vi "test_SessionsUnregistered_ReserveSessions_IndicatesSessionsDoNotExist.vi"(8 "error in":errorcluster) -> (0 "error out":errorcluster, 2 "result":string, 3 "pass":bool)   [LabVIEW 2020, in "MeasurementServerTests.lvlib" / "Session Reservation Tests.lvlib"]
uses:
  Session Reservation Tests.lvlib
  MeasurementServerTests.lvlib
  Runtime/Measurement Plugin Session Management V1/Session Reservation/Session Reservation.lvclass
  Runtime/Measurement Plugin Session Management Client/RPC Messages/ni_measurementlink_PinMapContext.ctl
  Runtime/Measurement Plugin Session Management Client/Measurement Plugin Session Management Client.lvlib
  Helpers/Pin Map XML Strings Global.vi
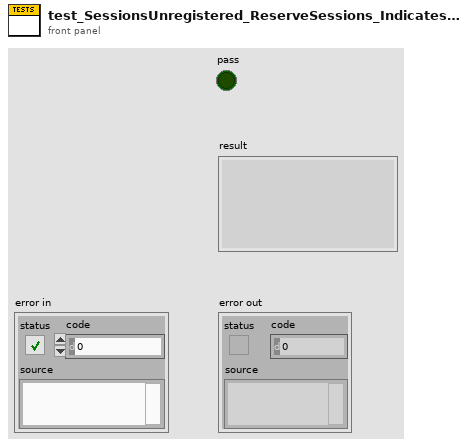
[diagram p1: front panel]
types:
  T1 = typedef "Measurement Plugin Session Management Client.lvlib/ni_measurementlink_PinMapContext.ctl" = cluster{"pin_map_id":string, "sites":i32[]}
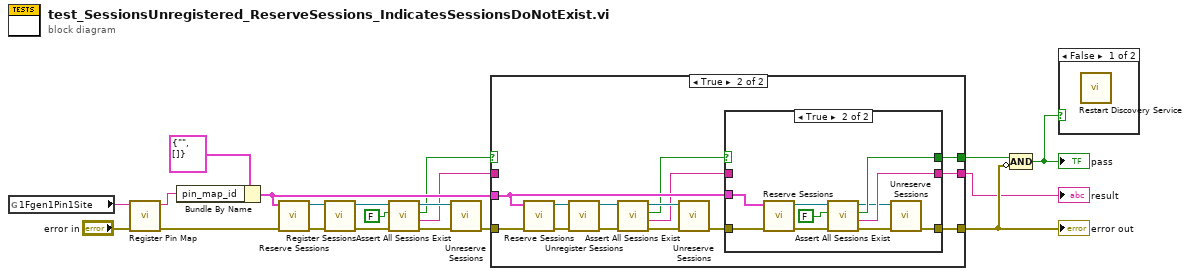
[diagram p0: block diagram]
diagram:
  n1 = global read "Pin Map XML Strings Global.vi" "1Fgen1Pin1Site"() -> (w17:string)
  n2 = call "Register Pin Map.vi"("error in"="error in", "pin map xml"=w17) -> ("error out"=w20:errorcluster, "pin map id"=w18:string)  [unwired: 8 in]
  n3 = Bundle By Name(cluster=T1 {"pin_map_id"="", "sites"=[]} ("pin map context"), "pin_map_id"=w18) -> (w10:T1)
  n4 = call "Reserve Sessions.vi"("error in"=w20, "pin map context"=w10) -> ("error out"=w15:errorcluster, "session reservation out"=w14:refnum<class "Session Reservation.lvclass">)  [unwired: 8 in]
  n5 = call "Register Sessions.vi"("error in"=w15, "session reservation in"=w14) -> ("error out"=w9:errorcluster, "session reservation out"=w7:refnum<class "Session Reservation.lvclass">)  [unwired: 8 in]
  n6 = call "Assert All Sessions Exist.vi"("error in"=w9, "expected value"=FALSE, "session reservation in"=w7) -> ("error out"=w8:errorcluster, "result"=w3:string, "pass"=w4:bool, "session reservation out"=w6:refnum<class "Session Reservation.lvclass">)  [unwired: 5 in]
  n7 = call "Unreserve Sessions.vi"("error in"=w8, "session reservation in"=w6) -> ("error out"=w11:errorcluster)  [unwired: 9 in]
  n8 = case shown="True" w4 {
    selector: w4 -> [w22 _]
    tunnel: [w23 w37] -> w13
    tunnel: w11 -> [w23 w36]
    tunnel: w10 -> [_ w35]
    tunnel: [w22 w25] -> w2
    tunnel: [w21 w24] -> w1
    tunnel: w3 -> [w21 _]
    frame False {
    }
    frame True {
      n9 = call "Reserve Sessions.vi"("error in"=w36, "pin map context"=w35) -> ("error out"=w34:errorcluster, "session reservation out"=w33:refnum<class "Session Reservation.lvclass">)  [unwired: 8 in]
      n10 = call "Unregister Sessions.vi"("error in"=w34, "session reservation in"=w33) -> ("error out"=w31:errorcluster, "session reservation out"=w29:refnum<class "Session Reservation.lvclass">)  [unwired: 8 in]
      n11 = call "Assert All Sessions Exist.vi"("error in"=w31, "session reservation in"=w29) -> ("error out"=w30:errorcluster, "result"=w26:string, "pass"=w27:bool, "session reservation out"=w28:refnum<class "Session Reservation.lvclass">)  [unwired: 6 in]
      n12 = call "Unreserve Sessions.vi"("error in"=w30, "session reservation in"=w28) -> ("error out"=w32:errorcluster)  [unwired: 9 in]
      n13 = case shown="True" w27 {
        selector: w27 -> [w40 _]
        tunnel: [w38 w50] -> w37
        tunnel: w35 -> [_ w49]
        tunnel: w32 -> [w38 w48]
        tunnel: w26 -> [w39 _]
        tunnel: [w40 w44] -> w25
        tunnel: [w39 w43] -> w24
        frame False {
        }
        frame True {
          n14 = call "Reserve Sessions.vi"("error in"=w48, "pin map context"=w49) -> ("error out"=w47:errorcluster, "session reservation out"=w46:refnum<class "Session Reservation.lvclass">)  [unwired: 8 in]
          n15 = call "Assert All Sessions Exist.vi"("error in"=w47, "expected value"=FALSE, "session reservation in"=w46) -> ("error out"=w41:errorcluster, "result"=w43:string, "pass"=w44:bool, "session reservation out"=w42:refnum<class "Session Reservation.lvclass">)  [unwired: 5 in]
          n16 = call "Unreserve Sessions.vi"("error in"=w41, "session reservation in"=w42) -> ("error out"=w50:errorcluster)  [unwired: 9 in]
        }
      }
    }
  }
  "error out" <- w13
  "result" <- w1
  n17 = Compound Arithmetic op=AND(w2, invert w13) -> (w12:bool)
  "pass" <- w12
  n18 = case shown="False" w12 {
    frame False {
      n19 = call "Restart Discovery Service.vi"() -> ()  [unwired: 11 in, 1 out]
    }
    frame True {
    }
  }
